vi "output_image.vi"(8 "error in (no error)":errorcluster, 11 "Graph_ref_in":refnum<vi>) -> (0 "error out":errorcluster, 3 "reference out":refnum<vi>)   [LabVIEW 2020, in "GraphBG_manage.lvlib" / "Graph.lvclass"]
uses:
  Graph.lvclass
  T50/subVI/xyY_graph.ctl
panel:
  out "new picture":picture
  in  "subset rect":T1
  in  "Path":path=path "C:/T50/jpg/xyY.png"
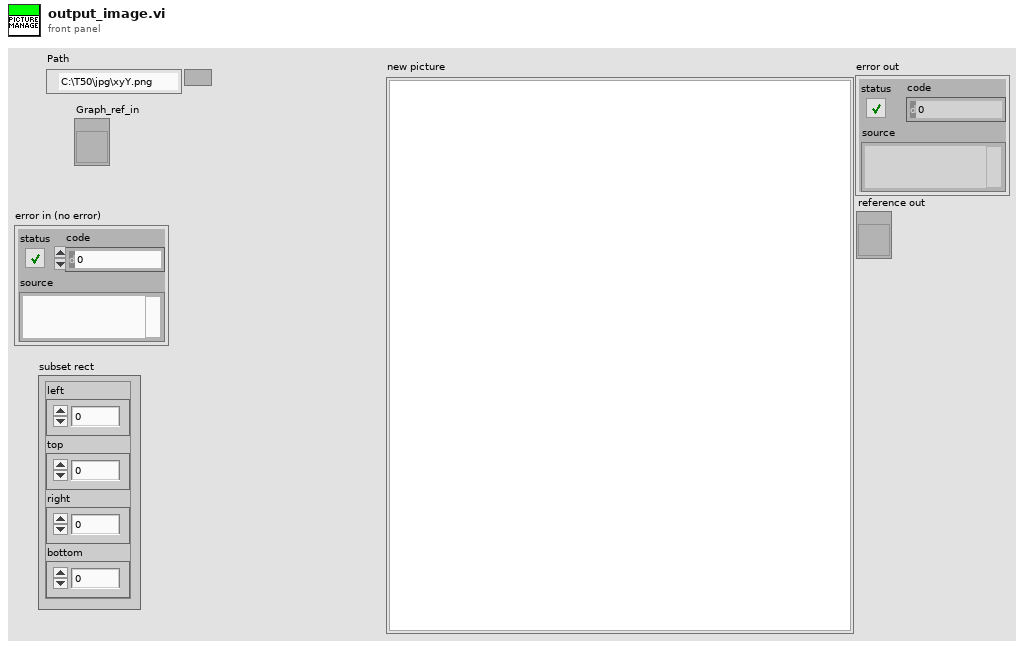
[diagram p1: front panel]
types:
  T1 = cluster{"left":i16, "top":i16, "right":i16, "bottom":i16}
  T2 = typedef "imagedata.ctl" = cluster{"image type":i32, "image depth":i32, "image":u8[], "mask":u8[], "colors":u32[], "Rectangle":cluster{"left":i16, "top":i16, "right":i16, "bottom":i16}}
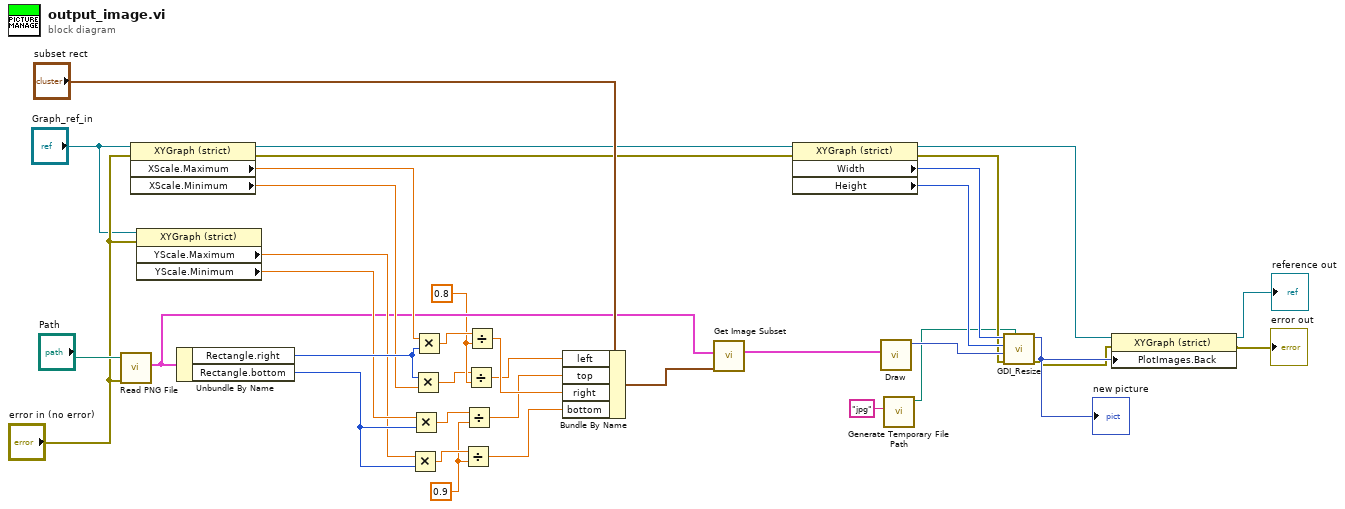
[diagram p0: block diagram]
diagram:
  w12 = 0.9 ("x")
  w15 = 0.8 ("x")
  n1 = call <vilib>:"Read PNG File.vi"("error in (no error)"="error in (no error)", "path to PNG file"="Path") -> ("image data"=w22:T2)  [unwired: 7 in, 2 out]
  n2 = property class="XYGraph (strict)"(reference="Graph_ref_in", error in="error in (no error)") -> (reference out=w9:refnum<vi>, error out=w10:errorcluster, "XScale.Maximum"=w34:dbl, "XScale.Minimum"=w29:dbl)
  n3 = property class="XYGraph (strict)"(reference="Graph_ref_in", error in="error in (no error)") -> ("YScale.Maximum"=w24:dbl, "YScale.Minimum"=w27:dbl)  [unwired: 2 out]
  n4 = Unbundle By Name(w22) -> ("Rectangle.right"=w30:i16, "Rectangle.bottom"=w28:i16)
  n5 = Multiply(x=w24, y=w28) -> (x*y=w13:dbl)
  n6 = Multiply(x=w27, y=w28) -> (x*y=w11:dbl)
  n7 = Multiply(x=w30, y=w29) -> (x*y=w14:dbl)
  n8 = Multiply(x=w34, y=w30) -> (x*y=w16:dbl)
  n9 = Divide(x=w13, y=w12) -> (x/y=w25:dbl)
  n10 = Divide(x=w11, y=w12) -> (x/y=w26:dbl)
  n11 = Divide(x=w14, y=w15) -> (x/y=w31:dbl)
  n12 = Divide(x=w16, y=w15) -> (x/y=w32:dbl)
  n13 = Bundle By Name(cluster="subset rect", "left"=w31, "top"=w26, "right"=w32, "bottom"=w25) -> (w23:T1)
  n14 = call <vilib>:"Get Image Subset.vi"("subset rect"=w23, "image data"=w22) -> ("image subset"=w21:T2)  [unwired: 4 in, 1 out]
  n15 = property class="XYGraph (strict)"(reference=w9, error in=w10) -> (reference out=w3:refnum<vi>, error out=w8:errorcluster, "Width"=w18:u32, "Height"=w19:u32)
  n16 = call "Draw.vi"("image data"=w21) -> ("new picture"=w17:picture)  [unwired: 8 in]
  n17 = call <vilib>:"Generate Temporary File Path.vi"("Temporary File Extension (tmp)"="jpg") -> ("Unique Temporary File Path"=w6:path)  [unwired: 9 in, 1 out]
  n18 = call "GDI_Resize.vi"("filename"=w6, "error in (no error)"=w8, "old image"=w17, "height"=w19, "width"=w18) -> ("error out"=w4:errorcluster, "new picture"=w5:picture)  [unwired: 5 in]
  "new picture" <- w5
  n19 = property class="XYGraph (strict)"(reference=w3, error in=w4, "PlotImages.Back"=w5) -> (reference out=→"reference out":refnum<vi>, error out=→"error out":errorcluster)
